vi "Handle_Custom_Content_Options.vi"(8 "error in (no error)":errorcluster, 11 "custom contents options":T1 {"list of controls options"."list which controls?" items=["all controls", "connected controls"]}) -> (0 "error out":errorcluster, 3 "previous custom contents options":T1 {"list of controls options"."list which controls?" items=["all controls", "connected controls"]})   [LabVIEW 2017, in "NI_ReportGenerationCore.lvlib"]
uses:
  <vilib>/Utility/NIReport.llb/NI_ReportGenerationCore.lvlib
  <vilib>/printing/EasyPrintingControls.llb/custom_contents_options.ctl
  <vilib>/printing/EasyPrintingControls.llb/list_which_controls.ctl
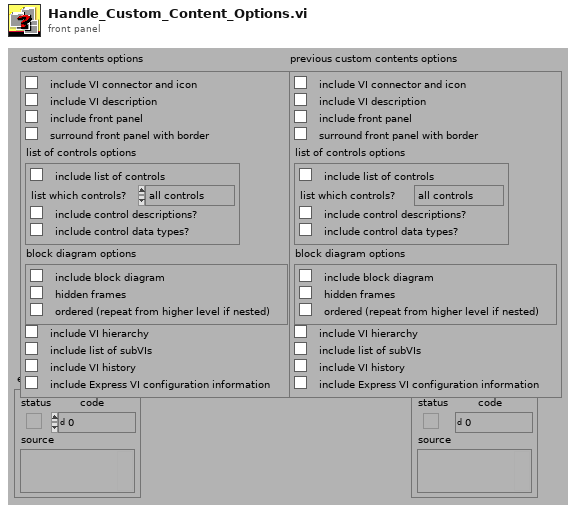
[diagram p1: front panel]
types:
  T1 = typedef "NI_ReportGenerationCore.lvlib/custom_contents_options.ctl" = cluster{"include VI connector and icon":bool, "include VI description":bool, "include front panel":bool, "surround front panel with border":bool, "list of controls options":cluster{"include list of controls":bool, "list which controls?":T2, "include control descriptions?":bool, "include control data types?":bool}, "block diagram options":cluster{"include block diagram":bool, "hidden frames":bool, "ordered (repeat from higher level if nested)":bool}, "include VI hierarchy":bool, "include list of subVIs":bool, "include VI history":bool, "include Express VI configuration information":bool}
  T2 = typedef "NI_ReportGenerationCore.lvlib/list_which_controls.ctl" = u16
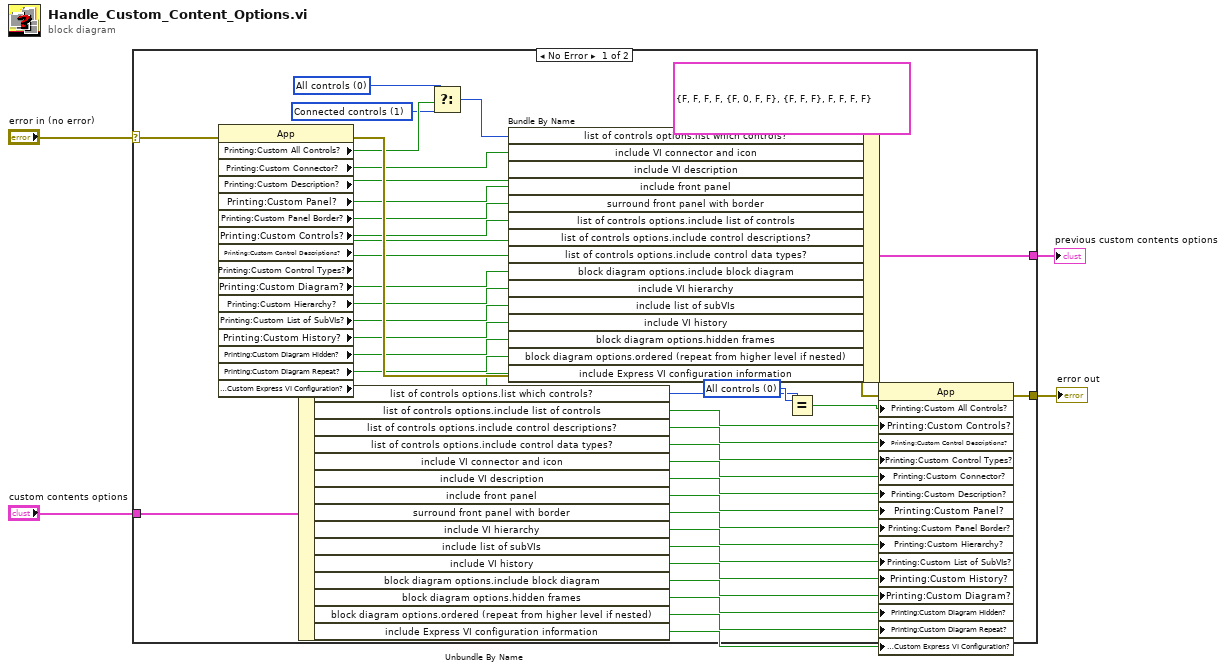
[diagram p0: block diagram]
diagram:
  n1 = case shown="No Error" "error in (no error)" {
    selector: "error in (no error)" -> [w41 w46]
    tunnel: [w6 w46] -> w3
    tunnel: [w39 _] -> w2
    tunnel: "custom contents options" -> [w5 _]
    frame No Error {
      w36 = T2 1 items=["All controls", "Connected controls"] ("List which controls?")
      w38 = T2 0 items=["All controls", "Connected controls"] ("List which controls?")
      w44 = T2 0 items=["All controls", "Connected controls"] ("List which controls?")
      n2 = property class="App"(error in=w41) -> (error out=w45:errorcluster, "Printing:Custom All Controls?"=w37:bool, "Printing:Custom Connector?"=w35:bool, "Printing:Custom Description?"=w29:bool, "Printing:Custom Panel?"=w28:bool, "Printing:Custom Panel Border?"=w26:bool, "Printing:Custom Controls?"=w27:bool, "Printing:Custom Control Descriptions?"=w31:bool, "Printing:Custom Control Types?"=w30:bool, "Printing:Custom Diagram?"=w34:bool, "Printing:Custom Hierarchy?"=w33:bool, "Printing:Custom List of SubVIs?"=w24:bool, "Printing:Custom History?"=w25:bool, "Printing:Custom Diagram Hidden?"=w11:bool, "Printing:Custom Diagram Repeat?"=w12:bool, "Printing:Custom Express VI Configuration?"=w8:bool)  [unwired: 1 in, 1 out]
      n3 = Unbundle By Name(w5) -> ("list of controls options.list which controls?"=w22:T2, "list of controls options.include list of controls"=w21:bool, "list of controls options.include control descriptions?"=w20:bool, "list of controls options.include control data types?"=w19:bool, "include VI connector and icon"=w43:bool, "include VI description"=w42:bool, "include front panel"=w18:bool, "surround front panel with border"=w17:bool, "include VI hierarchy"=w14:bool, "include list of subVIs"=w16:bool, "include VI history"=w15:bool, "block diagram options.include block diagram"=w13:bool, "block diagram options.hidden frames"=w10:bool, "block diagram options.ordered (repeat from higher level if nested)"=w9:bool, "include Express VI configuration information"=w7:bool)
      n4 = Select(t=w38, s=w37, f=w36) -> (s? t:f=w32:T2)
      n5 = Bundle By Name(cluster=T1 {"include VI connector and icon"=FALSE, "include VI description"=FALSE, "include front panel"=FALSE, "surround front panel with border"=FALSE, "list of controls options"={"include list of controls"=FALSE, "list which controls?"=0, "include control descriptions?"=FALSE, "include control data types?"=FALSE}, "block diagram options"={"include block diagram"=FALSE, "hidden frames"=FALSE, "ordered (repeat from higher level if nested)"=FALSE}, "include VI hierarchy"=FALSE, "include list of subVIs"=FALSE, "include VI history"=FALSE, "include Express VI configuration information"=FALSE} ("previous custom contents options"), "list of controls options.list which controls?"=w32, "include VI connector and icon"=w35, "include VI description"=w29, "include front panel"=w28, "surround front panel with border"=w26, "list of controls options.include list of controls"=w27, "list of controls options.include control descriptions?"=w31, "list of controls options.include control data types?"=w30, "block diagram options.include block diagram"=w34, "include VI hierarchy"=w33, "include list of subVIs"=w24, "include VI history"=w25, "block diagram options.hidden frames"=w11, "block diagram options.ordered (repeat from higher level if nested)"=w12, "include Express VI configuration information"=w8) -> (w39:T1)
      n6 = Equal?(x=w44, y=w22) -> (x = y?=w23:bool)
      n7 = property class="App"(error in=w45, "Printing:Custom All Controls?"=w23, "Printing:Custom Controls?"=w21, "Printing:Custom Control Descriptions?"=w20, "Printing:Custom Control Types?"=w19, "Printing:Custom Connector?"=w43, "Printing:Custom Description?"=w42, "Printing:Custom Panel?"=w18, "Printing:Custom Panel Border?"=w17, "Printing:Custom Hierarchy?"=w14, "Printing:Custom List of SubVIs?"=w16, "Printing:Custom History?"=w15, "Printing:Custom Diagram?"=w13, "Printing:Custom Diagram Hidden?"=w10, "Printing:Custom Diagram Repeat?"=w9, "Printing:Custom Express VI Configuration?"=w7) -> (error out=w6:errorcluster)  [unwired: 1 in, 1 out]
    }
    frame Error {
    }
  }
  "error out" <- w3
  "previous custom contents options" <- w2
